vi "Basic Move.vi"(0 "Velocity (mm/s)":dbl, 1 "Move size (um)":dbl, 2 "Move = True":bool, 3 "Feedback E.T.A":dbl, 4 "handle":i32, 5 "Axis":enum16{"M1", "M2", "M3"}(ring), 6 "Feedback Moving":bool) -> (7 "E.T.A.":dbl, 8 "Moving = False":bool)   [LabVIEW 2020]
uses:
  MicroDrive.dll
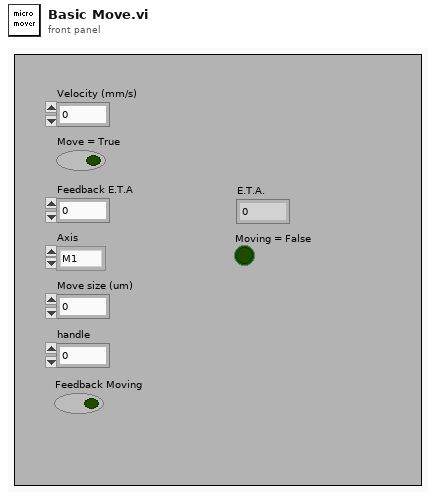
[diagram p1: front panel]
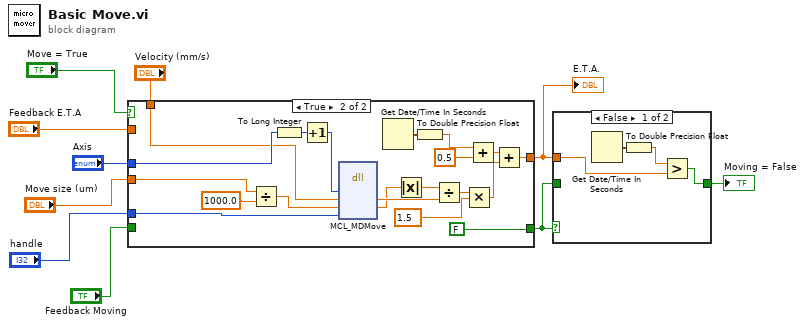
[diagram p0: block diagram]
diagram:
  n1 = case shown="True" "Move = True" {
    tunnel: "handle" -> [_ w20]
    tunnel: [w12 FALSE] -> w10
    tunnel: "Feedback Moving" -> [w12 _]
    tunnel: [w11 w25] -> w9
    tunnel: "Feedback E.T.A" -> [w11 _]
    tunnel: "Move size (um)" -> [_ w18]
    tunnel: "Axis" -> [_ w17]
    tunnel: "Velocity (mm/s)" -> [_ w16]
    frame False {
    }
    frame True {
      n2 = Divide(x=w18, y=1000.0) -> (x/y=w31:dbl)
      n3 = To Long Integer(number=w17) -> (32bit integer=w22:i32)
      n4 = Increment(x=w22) -> (x+1=w21:i32)
      n5 = dll-call lib="C:/Users/WalsworthGroup/Documents/Mad City Labs/MicroDrive/Labview Examples/MicroDrive.dll" fn="MCL_MDMove"("axis"=w21, "velocity"=w16, "distance"=w31, "handle"=w20) -> ("velocity"=w29:dbl, "distance"=w24:dbl)  [unwired: 5 in, 3 out]
      n6 = Get Date/Time In Seconds() -> (seconds since 1Jan1904=w19:timestamp)
      n7 = Absolute Value(x=w24) -> (abs(x)=w23:dbl)
      n8 = To Double Precision Float(number=w19) -> (double precision float=w14:dbl)
      n9 = Divide(x=w23, y=w29) -> (x/y=w28:dbl)
      n10 = Multiply(x=w28, y=1.5) -> (x*y=w26:dbl)
      n11 = Add(x=w14, y=0.5) -> (x+y=w15:dbl)
      n12 = Add(x=w15, y=w26) -> (x+y=w25:dbl)
    }
  }
  "E.T.A." <- w9
  n13 = case shown="False" w10 {
    tunnel: w10 -> [_ w37]
    tunnel: [w35 w37] -> w8
    tunnel: w9 -> [w34 _]
    frame False {
      n14 = Get Date/Time In Seconds() -> (seconds since 1Jan1904=w33:timestamp)
      n15 = To Double Precision Float(number=w33) -> (double precision float=w36:dbl)
      n16 = Greater?(x=w36, y=w34) -> (0:w35:bool)
    }
    frame True {
    }
  }
  "Moving = False" <- w8
